vi "Test App Get Deeply Nested Process by Qualified Name from Middle.vi"(8 "error in (no error)":errorcluster, 11 "Application Test in":refnum<class "Application Dev Test.lvclass">) -> (0 "error out":errorcluster, 3 "Application Test out":refnum<class "Application Dev Test.lvclass">)   [LabVIEW 2020, in "Application Dev Test.lvclass"]
uses:
  Application Dev Test.lvclass
  C:/Program Files (x86)/National Instruments/LabVIEW 2020/vi.lib/Astemes/LUnit/Test Case.lvclass
  source/Framework/Process/Process.lvclass
  source/Framework/Process/Process.lvclass/Process.ctl
  source/Framework/Application/Application.lvclass/Application.ctl
  <vilib>/Astemes/LUnit/Test Case.lvclass/Test Case.ctl
  source/Framework/Application/Private/Add Process to Map.vi
  source/Framework/Application/Private/Throw Error If Process Already in App.vi
  source/Framework/Process/Protected/Messaging/Send Message.vi
  source/Framework/Process/Public/Lifecycle/Get Lifecycle State.vi
  source/Framework/Process/Protected/SubVIs/Set Context.vi
  source/Framework/Application/Private/Retrieve Process from App.vi
  source/Framework/Application/Private/Parse Process Name.vi
  source/Framework/Application/Private/Get Process from Map.vi
  <vilib>/Astemes/LUnit/Palette/Pass.vi
  <vilib>/Astemes/LUnit/Palette/Fail.vi
  <vilib>/Astemes/LUnit/Set Assertion Type.vi
  source/Framework/Process/Private/SubVIs/Wait for finish.vi
  source/Framework/Process/Private/SubVIs/Set Lifecycle State.vi
  source/Framework/Process/Private/SubVIs/Handle Debug Data.vi
  <vilib>/Utility/error.llb/Clear Errors.vi
  source/Framework/Process/Public/Lifecycle/Leave Process Loop.vi
  source/Framework/Process/Protected/Messaging/Request Message.vi
  <vilib>/AdvancedString/Delimited String to 1D String Array.vi
  <vilib>/Astemes/LUnit/Add test result.vi
  source/Framework/Logging/Log Debug.vi
  <vilib>/AdvancedString/1D String Array to Delimited String.vi
  <vilib>/Utility/High Resolution Relative Seconds.vi
  source/Framework/Process/Private/SubVIs/Enqueue Request Message.vi
  <vilib>/Astemes/LUnit/LUnit Record Assertion Result.vi
  <vilib>/Astemes/LUnit/LUnit Aggregate Assertion Results.vi
  <vilib>/Astemes/LUnit/Method Result/LUnit Merge Status.vi
  <vilib>/Astemes/LUnit/LUnit Concatenate result strings.vi
  source/Framework/Application/Application.lvclass
  C:/Git/astemes-triarc-framework/source/Framework/Process/Process.lvclass
  <vilib>/Utility/error.llb/Error Cluster From Error Code.vi
  source/Framework/Process/Public/Read Name.vi
  source/Framework/Process/Private/SubVIs/Wait for Response Message.vi
  <vilib>/Astemes/LUnit/Test Case.lvclass
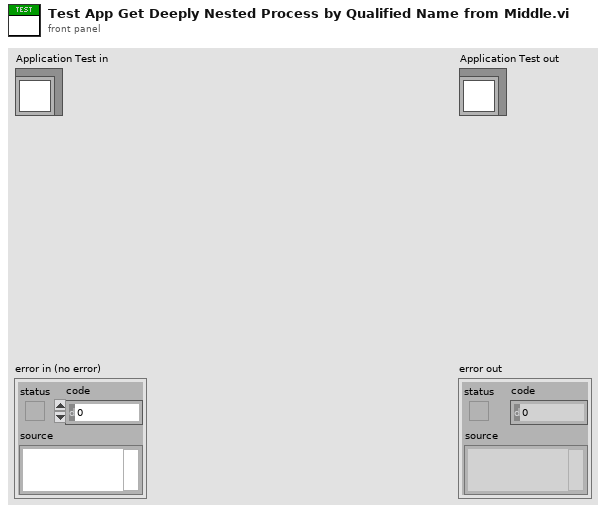
[diagram p1: front panel]
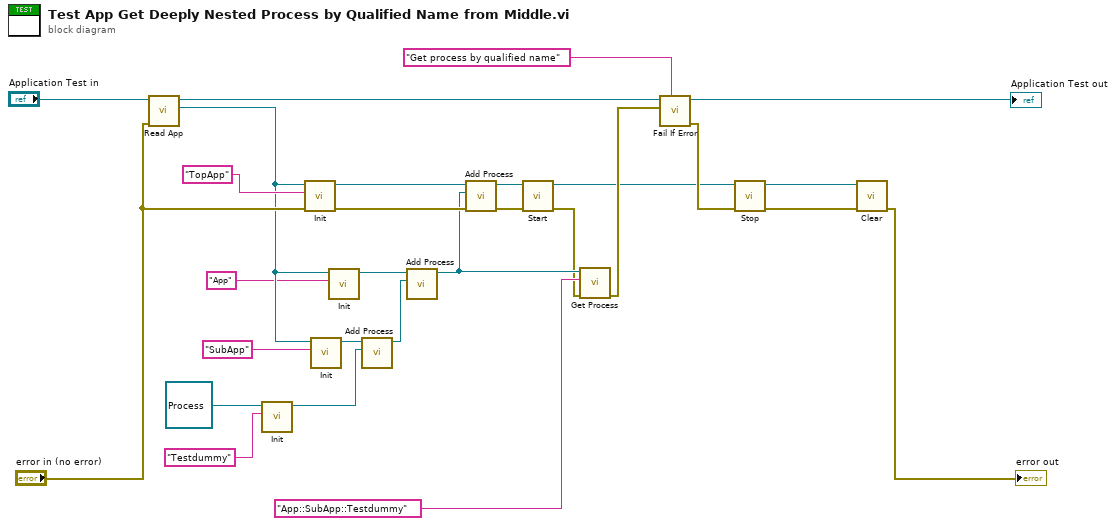
[diagram p0: block diagram]
diagram:
  n1 = call "Read App.vi"("error in (no error)"="error in (no error)", "Application Test In"="Application Test in") -> ("App out"=w11:refnum<class "Application.lvclass">, "Application Test Out"=w28:refnum<class "Application Dev Test.lvclass">)  [unwired: 7 in, 1 out]
  n2 = call-dynamic "Init.vi"("Name"="Testdummy", "Process In"=refnum<class "Process.lvclass"> refnum ("Process.lvclass")) -> ("Process Out"=w12:refnum<class "Process.lvclass">)  [unwired: 8 in, 1 out]
  n3 = call-dynamic "Init.vi"("error in (no error)"="error in (no error)", "Name"="TopApp", "Process In"=w11) -> ("error out"=w26:errorcluster, "Process Out"=w27:refnum<class "Application.lvclass">)  [unwired: 7 in]
  n4 = call-dynamic "Init.vi"("Name"="SubApp", "Process In"=w11) -> ("Process Out"=w13:refnum<class "Application.lvclass">)  [unwired: 8 in, 1 out]
  n5 = call-dynamic "Init.vi"("Name"="App", "Process In"=w11) -> ("Process Out"=w10:refnum<class "Application.lvclass">)  [unwired: 8 in, 1 out]
  n6 = call "Add Process.vi"("Process"=w12, "Application In"=w13) -> ("Application Out"=w9:refnum<class "Application.lvclass">)  [unwired: 8 in, 1 out]
  n7 = call "Add Process.vi"("Process"=w9, "Application In"=w10) -> ("Application Out"=w7:refnum<class "Application.lvclass">)  [unwired: 8 in, 1 out]
  n8 = call "Add Process.vi"("error in (no error)"=w26, "Process"=w7, "Application In"=w27) -> ("error out"=w6:errorcluster, "Application Out"=w2:refnum<class "Application.lvclass">)  [unwired: 7 in]
  n9 = call "Start.vi"("error in (no error)"=w6, "Process In"=w2) -> ("error out"=w3:errorcluster, "Process Out"=w1:refnum<class "Application.lvclass">)  [unwired: 7 in, 1 out]
  n10 = call "Get Process.vi"("error in (no error)"=w3, "Process Name"="App::SubApp::Testdummy" ("Name"), "Application In"=w7) -> ("error out"=w5:errorcluster)  [unwired: 6 in, 2 out]
  n11 = call <vilib>:"Fail If Error.vi"("Description"="Get process by qualified name", "Assert error"=w5, "LUnit Test Case In"=w28) -> ("error out"=w22:errorcluster, "LUnit Test Case Out"=→"Application Test out":refnum<class "Application Dev Test.lvclass">)  [unwired: 7 in]
  n12 = call "Stop.vi"("error in (no error)"=w22, "Process In"=w1) -> ("error out"=w19:errorcluster, "Process Out"=w25:refnum<class "Application.lvclass">)  [unwired: 7 in, 1 out]
  n13 = call-dynamic "Clear.vi"("error in (no error)"=w19, "Application In"=w25) -> ("error out"=→"error out":errorcluster)  [unwired: 9 in]
